vi "COM_Test.vi"() -> ()   [LabVIEW 2020]
uses:
  <vilib>/Instr/_visa.llb/VISA Configure Serial Port (Instr).vi
panel:
  in  "milliseconds to wait":u32
  in  "stop":bool
  out "concatenated string":string
  out "unsigned byte array":u8[](array[numeric])
  out "error out":errorcluster
  in  "error in (no error)":errorcluster
  in  "baud rate (9600)":u32=9600
  in  "VISA resource name":refnum<visa-resource-name>
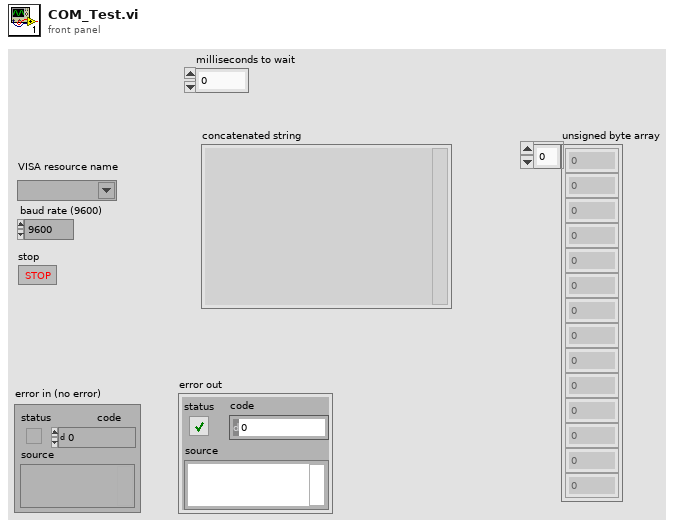
[diagram p1: front panel]
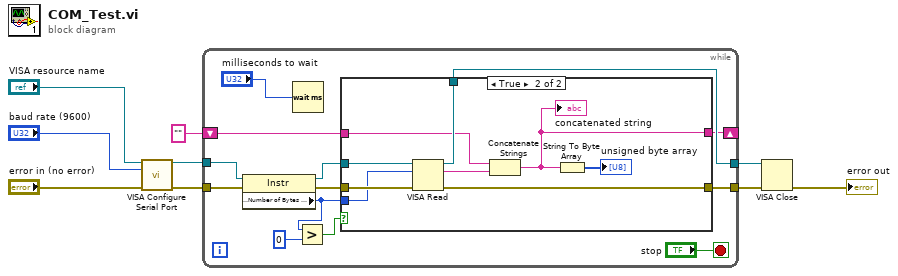
[diagram p0: block diagram]
diagram:
  n1 = call-poly "VISA Configure Serial Port"("VISA resource name"="VISA resource name", "baud rate (9600)"="baud rate (9600)", "error in (no error)"="error in (no error)") -> ("VISA resource name out"=w5:refnum<visa-resource-name>, "error out"=w6:errorcluster)  [unwired: 11 in]
  n2 = while {
    tunnel: w6 -> [w22]
    tunnel: w5 -> [w21]
    tunnel: [w18] -> w4
    tunnel: [w17] -> w3
    shift-right: [w14] -> _
    shift-left: "" -> [w13]
    stop <- "stop" stop-if-true
    n3 = property class="Instr"(reference=w21, error in=w22) -> (reference out=w20:refnum<visa-resource-name>, error out=w19:errorcluster, "Serial Settings:Number of Bytes at Serial Port"=w11:u32)
    n4 = Wait (ms)(milliseconds to wait="milliseconds to wait") -> ()  [unwired: 1 out]
    n5 = Greater?(x=w11, y=u32 0) -> (0:w12:bool)
    n6 = case shown="True" w12 {
      tunnel: w20 -> [w25 w34]
      tunnel: w19 -> [w23 w33]
      tunnel: w11 -> [_ w32]
      tunnel: [w23 w31] -> w18
      tunnel: [w25 w30] -> w17
      tunnel: [w24 w27] -> w14
      tunnel: w13 -> [w24 w26]
      frame False {
      }
      frame True {
        n7 = VISA Read(VISA resource name=w34, byte count=w32, error in (no error)=w33) -> (VISA resource name out=w30:refnum<visa-resource-name>, read buffer=w28:string, error out=w31:errorcluster)  [unwired: 1 out]
        n8 = Concatenate Strings(w26, w28) -> (w27:string)
        "concatenated string" <- w27
        n9 = String To Byte Array(string=w27) -> (unsigned byte array=→"unsigned byte array":u8[])
      }
    }
  }
  n10 = VISA Close(VISA resource name=w3, error in (no error)=w4) -> (error out=→"error out":errorcluster)
